vi "gun_turret_input_scale.vi"(10 "Voltage":dbl, 11 "Gun Const":T1={"gun"={"num_lines"=0.0, "gain_kp1"=0.0, "gain_kp2"=0.0, "gain_ki"=0.0, "gain_kd"=0.0}, "turret"={"center_ana"=0.0, "volts_per_180"=0.0, "man_scale"=0.0, "turret_idg"={"low_fault_ana"=0.0, "high_fault_ana"=0.0, "min_ana"=0.0, "max_ana"=0.0, "movement_thresh"=0.0, "movement_time"=0.0}, "turret_pid"={"kP"=0.0, "kI"=0.0, "kD"=0.0}, "turret_invert"=TRUE, "turret_low_power"=0.0}, "tracking"={"velocity_lead_gain"=0.0, "velocity_rotation_gain"=0.0}, "hood"={"hood_idg"={"low_fault_ana"=0.0, "high_fault_ana"=0.0, "min_ana"=0.0, "max_ana"=0.0, "movement_thresh"=0.0, "movement_time"=0.0}, "hood_pid"={"kP"=0.0, "kI"=0.0, "kD"=0.0}, "hood_scale"={"min_ana"=0.0, "min_units"=0.0, "max_ana"=0.0, "max_units"=0.0}, "hood_invert"=FALSE}}) -> (3 "Angle":dbl)   [LabVIEW 2011]
uses:
  gun_const_t.ctl
  gun_idg_const.ctl
  common/gain_const.ctl
  common/scale_const.ctl
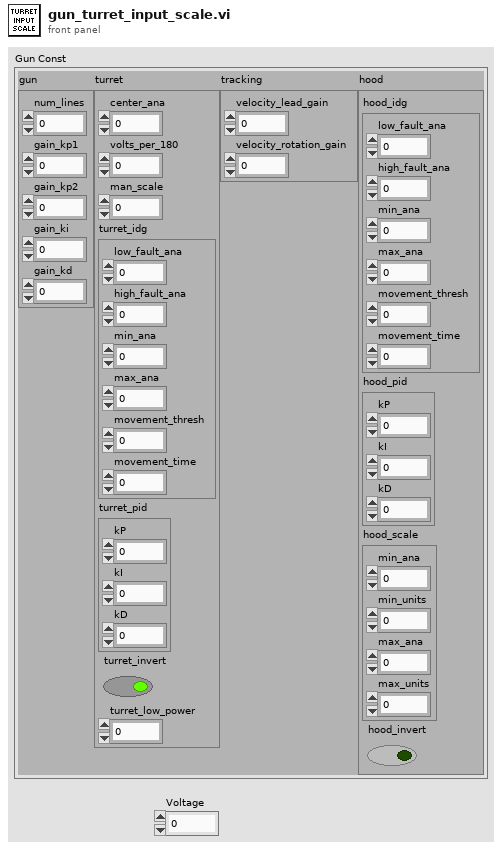
[diagram p1: front panel]
types:
  T1 = typedef "gun_const_t.ctl" = cluster{"gun":cluster{"num_lines":dbl, "gain_kp1":dbl, "gain_kp2":dbl, "gain_ki":dbl, "gain_kd":dbl}, "turret":cluster{"center_ana":dbl, "volts_per_180":dbl, "man_scale":dbl, "turret_idg":T2, "turret_pid":T3, "turret_invert":bool, "turret_low_power":dbl}, "tracking":cluster{"velocity_lead_gain":dbl, "velocity_rotation_gain":dbl}, "hood":cluster{"hood_idg":T2, "hood_pid":T3, "hood_scale":T4, "hood_invert":bool}}
  T2 = typedef "gun_idg_const.ctl" = cluster{"low_fault_ana":dbl, "high_fault_ana":dbl, "min_ana":dbl, "max_ana":dbl, "movement_thresh":dbl, "movement_time":dbl}
  T3 = typedef "gain_const.ctl" = cluster{"kP":dbl, "kI":dbl, "kD":dbl}
  T4 = typedef "scale_const.ctl" = cluster{"min_ana":dbl, "min_units":dbl, "max_ana":dbl, "max_units":dbl}
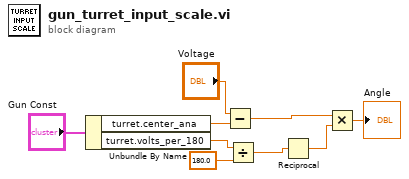
[diagram p0: block diagram]
diagram:
  n1 = Unbundle By Name("Gun Const") -> ("turret.center_ana"=w6:dbl, "turret.volts_per_180"=w4:dbl)
  n2 = Subtract(x="Voltage", y=w6) -> (x-y=w8:dbl)
  n3 = Divide(x=w4, y=180.0) -> (x/y=w1:dbl)
  n4 = Reciprocal(x=w1) -> (1/x=w2:dbl)
  n5 = Multiply(x=w8, y=w2) -> (x*y=→"Angle":dbl)
